vi "Chi-Squared CDF.vi"(10 "k":i32=1, 11 "x":dbl=1.0) -> (0 "error":i32, 3 "cdf(x)":dbl=0.682689492137086)   [LabVIEW 2017, in "NI_Gmath.lvlib"]
doc: "Computes the continuous cumulative distribution function (CDF), or the probability that the random variate X, where X describes the selected distribution type, has a value less than or equal to <B>x</B>. You must manually select the polymorphic instance to use."
uses:
  NI_Gmath.lvlib
  st_error_code.ctl
  Incomplete Gamma Function.vi
panel:
  # "Chi-Squared CDF"
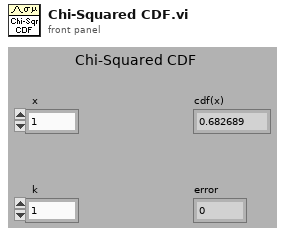
[diagram p1: front panel]
types:
  T1 = typedef "NI_Gmath.lvlib/st_error_code.ctl" = i32
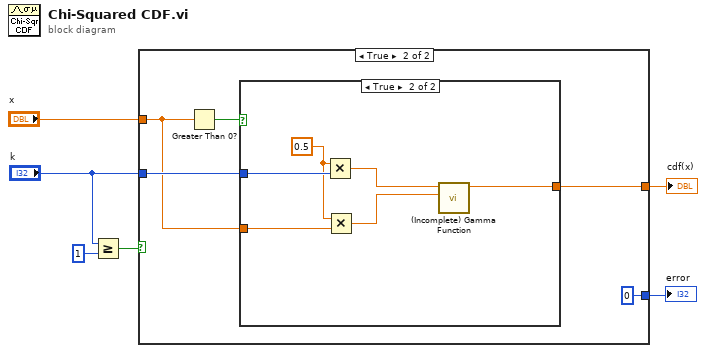
[diagram p0: block diagram]
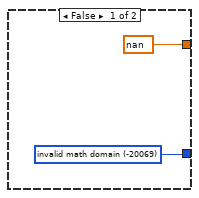
[diagram p2: hidden frame]
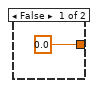
[diagram p3: hidden frame]
diagram:
  n1 = Greater Or Equal?(x="k", y=1) -> (x >= y?=w1:bool)
  n2 = case shown="True" w1 {
    tunnel: [w7 0 ("invalid math domain")] -> w6
    tunnel: [nan w12] -> w5
    tunnel: "x" -> [_ w10]
    tunnel: "k" -> [_ w11]
    frame False {
      w7 = T1 -20069 items=["invalid math domain"=-20069, "Fourier interpolation size m >= n"=-20070, "empty array"=-20003] ("stat interp error code")
    }
    frame True {
      n3 = Greater Than 0?(x=w10) -> (x > 0?=w9:bool)
      n4 = case shown="True" w9 {
        tunnel: [0.0 w16] -> w12
        tunnel: w10 -> [_ w18]
        tunnel: w11 -> [_ w20]
        frame False {
        }
        frame True {
          w17 = 0.5 ("x")
          n5 = Multiply(x=w17, y=w20) -> (x*y=w19:dbl)
          n6 = Multiply(x=w17, y=w18) -> (x*y=w15:dbl)
          n7 = call-poly "(Incomplete) Gamma Function.vi"("a"=w15, "x"=w19) -> ("g(x, a)"=w16:dbl)  [unwired: 9 in]
        }
      }
    }
  }
  "cdf(x)" <- w5
  "error" <- w6
